vi "Auton_S1_Left_Switch.vi"   [LabVIEW 2017]
uses:
  <vilib>/Rock Robotics/WPI/Utilities/WPI_GetSetVariantRefNum.vi
  Robot Global Data.vi
  <vilib>/Rock Robotics/WPI/RobotDrive/WPI_RobotDriveArcadeDrive_Standard(NoSaturation).vi
types:
  T1 = typedef "WPI_RobotDriveDevRef.ctl" = cluster{"DevStatus":errorcluster, "Motors[]":T2[], "Square Inputs":bool, "Max Output":dbl}
  T2 = typedef "WPI_MotorControlDeviceRef.ctl" = cluster{"DeviceStatus":errorcluster, "Type":T3, "PWM":cluster{"PWM Channel":T4, "DeadBand":T5}, "CAN":cluster{"Device Number":u8, "SetOutput VI Ref":variant, "GetOutput VI Ref":variant, "Enable VI Ref":variant, "Disable VI Ref":variant, "Data":variant}, "Invert":bool, "DIO PWM":cluster{"PWM \"Enable\" Channel":T4, "DIOChannel":T6, "PWM Rate":dbl}}
  T3 = typedef "WPI_MotorControlType.ctl" = enum16{"PWM", "CAN", "DIO PWM"}
  T4 = typedef "FPGA_DIOPWMChannel.ctl" = enum8{"PWM 0", "PWM 1", "PWM 2", "PWM 3", "PWM 4", "PWM 5", "PWM 6", "PWM 7", "PWM 8", "PWM 9", "PWM MXP 0", "PWM MXP 1", "PWM MXP 2", "PWM MXP 3", "PWM MXP 4", "PWM MXP 5", "PWM MXP 6", "PWM MXP 7", "PWM MXP 8", "PWM MXP 9", "Invalid"}
  T5 = typedef "WPI_PWMDeadband.ctl" = cluster{"Name":string, "maxPositivePwm":i32, "minPositivePwm":i32, "centerPwm":i32, "maxNegativePwm":i32, "minNegativePwm":i32, "angularRange":u16}
  T6 = typedef "FPGA_DIOChannel.ctl" = enum8{"DIO 0", "DIO 1", "DIO 2", "DIO 3", "DIO 4", "DIO 5", "DIO 6", "DIO 7", "DIO 8", "DIO 9", "DIO MXP 0", "DIO MXP 1", "DIO MXP 2", "DIO MXP 3", "DIO MXP 4", "DIO MXP 5", "DIO MXP 6", "DIO MXP 7", "DIO MXP 8", "DIO MXP 9", "DIO MXP 10", "DIO MXP 11", "DIO MXP 12", "DIO MXP 13", "DIO MXP 14", "DIO MXP 15", "SPI Port CS1", "SPI Port CS2", "SPI Port CS3", "SPI Port MISO", "SPI Port MOSI", "Invalid"}
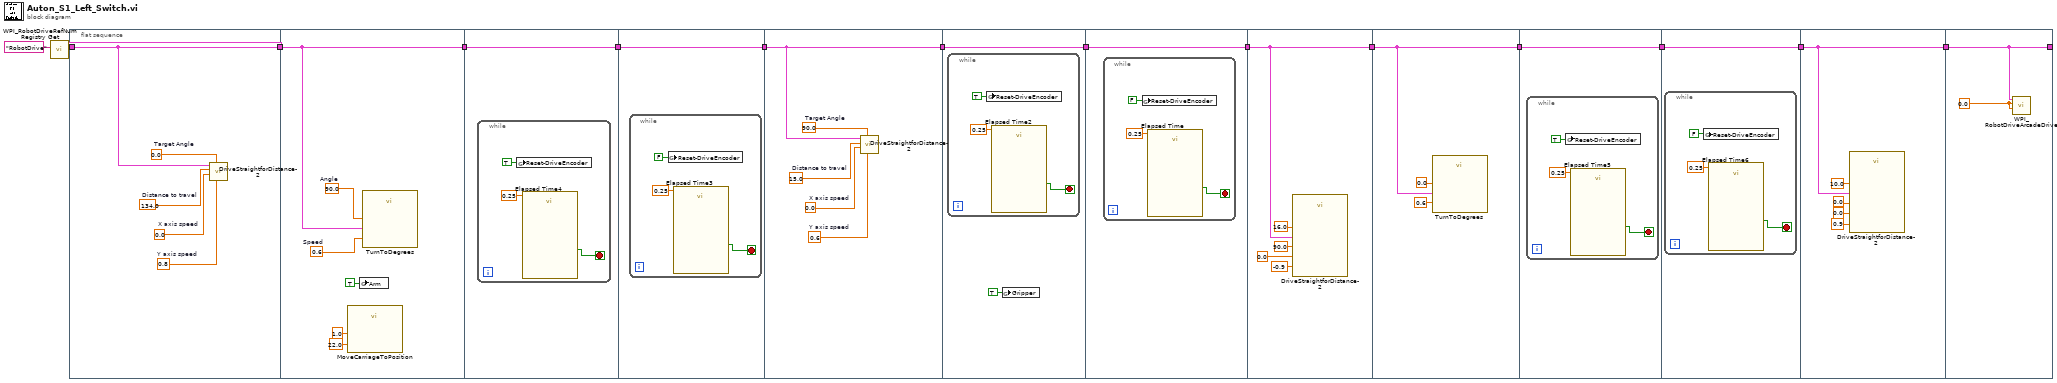
[diagram p0: block diagram]
diagram:
  n1 = call <vilib>:"WPI_RobotDriveRefNum Registry Get.vi"("refnum name"="RobotDrive") -> ("RobotDriveDevRef"=w13:T1)  [unwired: 9 in, 1 out]
  n2 = flat-sequence {
    tunnel: [w19] -> w9
    tunnel: w13 -> [w19]
    tunnel: w9 -> [w24]
    tunnel: [w24] -> w8
    tunnel: w8 -> [w26]
    tunnel: [w26] -> w10
    tunnel: w10 -> [w30]
    tunnel: [w30] -> w11
    tunnel: w11 -> [w34]
    tunnel: [w34] -> w12
    tunnel: w12 -> [w40]
    tunnel: [w40] -> w6
    tunnel: w6 -> [w44]
    tunnel: [w44] -> w5
    tunnel: w5 -> [w52]
    tunnel: [w52] -> w7
    tunnel: w7 -> [w55]
    tunnel: [w55] -> w3
    tunnel: w3 -> [w56]
    tunnel: [w56] -> w2
    tunnel: w2 -> [w60]
    tunnel: [w60] -> w1
    tunnel: w1 -> [w67]
    tunnel: [w67] -> w4
    tunnel: [w69] -> _
    tunnel: w4 -> [w69]
    frame #0 {
      w15 = 0.0  # Target Angle
      w16 = 0.8  # Y axis speed
      w17 = 0.0  # X axis speed
      w18 = 134.0  # Distance to travel
      n3 = call "DriveStraightforDistance-2.vi"("Y axis speed"=w16, "Target Angle"=w15, "X axis speed"=w17, "Distance to travel"=w18, "RobotDriveDevRef"=w19) -> ()  [unwired: 7 in]
    }
    frame #1 {
      w23 = 90.0  # Angle
      w25 = 0.6  # Speed
      n4 = call "MoveCarriageToPosition.vi"("Lift Speed"=1.0, "Target Height"=22.0) -> ()  [unwired: 10 in]
      n5 = global write "Robot Global Data.vi" "Arm"(TRUE ("Arm")) -> ()
      n6 = call "TurnToDegrees.vi"("Speed"=w25, "RobotDriveDevRef"=w24, "Angle"=w23) -> ()  [unwired: 9 in]
    }
    frame #2 {
      n7 = while {
        stop <- w29 stop-if-true
        n8 = global write "Robot Global Data.vi" "Reset-DriveEncoder"(TRUE ("Reset-DriveEncoder")) -> ()
        n9 = call "Elapsed Time4"("Time Target (s)"=0.25) -> ("Time has Elapsed"=w29:bool)  [unwired: 11 in, 7 out]
      }
    }
    frame #3 {
      n10 = while {
        stop <- w33 stop-if-true
        n11 = global write "Robot Global Data.vi" "Reset-DriveEncoder"(FALSE ("Reset-DriveEncoder")) -> ()
        n12 = call "Elapsed Time3"("Time Target (s)"=0.25) -> ("Time has Elapsed"=w33:bool)  [unwired: 11 in, 7 out]
      }
    }
    frame #4 {
      w35 = 90.0  # Target Angle
      w36 = 0.6  # Y axis speed
      w37 = 0.0  # X axis speed
      w38 = 15.0  # Distance to travel
      n13 = call "DriveStraightforDistance-2.vi"("Y axis speed"=w36, "Target Angle"=w35, "X axis speed"=w37, "Distance to travel"=w38, "RobotDriveDevRef"=w34) -> ()  [unwired: 7 in]
    }
    frame #5 {
      n14 = while {
        stop <- w43 stop-if-true
        n15 = global write "Robot Global Data.vi" "Reset-DriveEncoder"(TRUE ("Reset-DriveEncoder")) -> ()
        n16 = call "Elapsed Time2"("Time Target (s)"=0.25) -> ("Time has Elapsed"=w43:bool)  [unwired: 11 in, 7 out]
      }
      n17 = global write "Robot Global Data.vi" "Gripper"(TRUE ("Gripper")) -> ()
    }
    frame #6 {
      n18 = while {
        stop <- w47 stop-if-true
        n19 = global write "Robot Global Data.vi" "Reset-DriveEncoder"(FALSE ("Reset-DriveEncoder")) -> ()
        n20 = call "Elapsed Time"("Time Target (s)"=0.25) -> ("Time has Elapsed"=w47:bool)  [unwired: 11 in, 7 out]
      }
    }
    frame #7 {
      n21 = call "DriveStraightforDistance-2.vi"("Y axis speed"=-0.9, "Target Angle"=90.0, "X axis speed"=0.0, "Distance to travel"=16.0, "RobotDriveDevRef"=w52) -> ()  [unwired: 7 in]
    }
    frame #8 {
      n22 = call "TurnToDegrees.vi"("Speed"=0.6, "RobotDriveDevRef"=w55, "Angle"=0.0) -> ()  [unwired: 9 in]
    }
    frame #9 {
      n23 = while {
        stop <- w59 stop-if-true
        n24 = global write "Robot Global Data.vi" "Reset-DriveEncoder"(TRUE ("Reset-DriveEncoder")) -> ()
        n25 = call "Elapsed Time5"("Time Target (s)"=0.25) -> ("Time has Elapsed"=w59:bool)  [unwired: 11 in, 7 out]
      }
    }
    frame #10 {
      n26 = while {
        stop <- w63 stop-if-true
        n27 = global write "Robot Global Data.vi" "Reset-DriveEncoder"(FALSE ("Reset-DriveEncoder")) -> ()
        n28 = call "Elapsed Time6"("Time Target (s)"=0.25) -> ("Time has Elapsed"=w63:bool)  [unwired: 11 in, 7 out]
      }
    }
    frame #11 {
      n29 = call "DriveStraightforDistance-2.vi"("Y axis speed"=0.9, "Target Angle"=0.0 ("Y axis speed"), "X axis speed"=0.0, "Distance to travel"=10.0, "RobotDriveDevRef"=w67) -> ()  [unwired: 7 in]
    }
    frame #12 {
      w70 = 0.0 ("X axis value")
      n30 = call-poly <vilib>:"WPI_RobotDriveArcadeDrive.vi"("Y axis value"=w70, "X axis value"=w70, "RobotDriveDevRef"=w69) -> ()  [unwired: 6 in, 3 out]
    }
  }
